vi "Page_Dialog_Write.vi"(6 "ctlReferences":T1, 8 "error in (no error)":errorcluster, 11 "Class in":refnum<class "Installer.lvclass">) -> (0 "error out":errorcluster, 3 "Class out":refnum<class "Installer.lvclass">)   [LabVIEW 2020, in "Installer.lvclass"]
uses:
  <vilib>/AppBuilder/IB_Classes/Installer/Installer.lvclass
  <resource>/Framework/Providers/Builds/Installer/Pages/controls/IB_UI_Page_Dialog_Info_References.ctl
  <resource>/Framework/Providers/Builds/Installer/CDK_sTypeDef_Languages.ctl
  <resource>/Framework/Providers/Common/provcom_BrowseProjectFile2.ctl
  <vilib>/AppBuilder/IB_Classes/Installer/Installer.lvclass/Installer.ctl
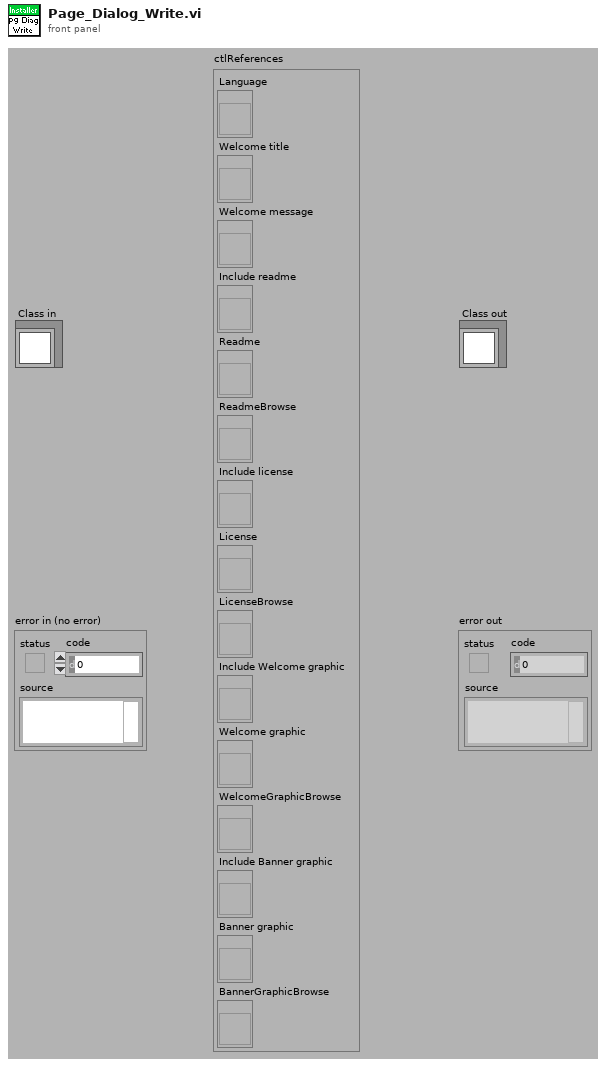
[diagram p1: front panel]
types:
  T1 = typedef "IB_UI_Page_Dialog_Info_References.ctl" = cluster{"Language":refnum<vi>, "Welcome title":refnum<vi>, "Welcome message":refnum<vi>, "Include readme":refnum<vi>, "Readme":refnum<vi>, "ReadmeBrowse":refnum<vi>, "Include license":refnum<vi>, "License":refnum<vi>, "LicenseBrowse":refnum<vi>, "Include Welcome graphic":refnum<vi>, "Welcome graphic":refnum<vi>, "WelcomeGraphicBrowse":refnum<vi>, "Include Banner graphic":refnum<vi>, "Banner graphic":refnum<vi>, "BannerGraphicBrowse":refnum<vi>}
  T2 = typedef "CDK_sTypeDef_Languages.ctl" = u16
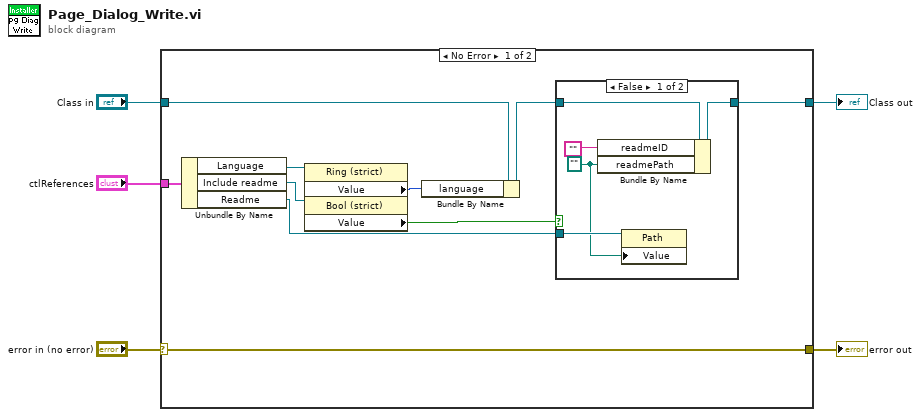
[diagram p0: block diagram]
diagram:
  n1 = case shown="No Error" "error in (no error)" {
    selector: "error in (no error)" -> [w11 w23]
    tunnel: [w11 w23] -> w4
    tunnel: [w8 w22] -> w2
    tunnel: "Class in" -> [w13 w22]
    tunnel: "ctlReferences" -> [w15 _]
    frame No Error {
      n2 = Unbundle By Name(w15) -> ("Language"=w12:refnum<vi>, "Include readme"=w14:refnum<vi>, "Readme"=w6:refnum<vi>)
      n3 = property class="Ring (strict)"(reference=w12) -> ("Value"=w10:T2)  [unwired: 1 in, 2 out]
      n4 = property class="Bool (strict)"(reference=w14) -> ("Value"=w7:bool)  [unwired: 1 in, 2 out]
      n5 = Bundle By Name(cluster=w13, "language"=w10) -> (w9:refnum<class "Installer.lvclass">)
      n6 = case shown="False" w7 {
        tunnel: [w19 w21] -> w8
        tunnel: w9 -> [w20 w21]
        tunnel: w6 -> [w17 _]
        frame False {
          w16 = path ""
          n7 = Bundle By Name(cluster=w20, "readmeID"="", "readmePath"=w16) -> (w19:refnum<class "Installer.lvclass">)
          n8 = property class="Path"(reference=w17, "Value"=w16) -> ()  [unwired: 1 in, 2 out]
        }
        frame True {
        }
      }
    }
    frame Error {
    }
  }
  "error out" <- w4
  "Class out" <- w2
